vi "GetOneProperty.vi"() -> (0 "error out":errorcluster={"status"=TRUE, "code"=-375006, "source"="Unflatten From JSON in GetOneProperty.vi"}, 3 "setflag":string)   [LabVIEW 2019]
uses:
  <vilib>/httpClient/LabVIEWHTTPClient.lvlib
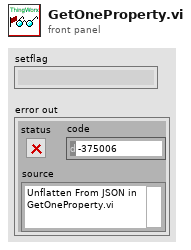
[diagram p1: front panel]
types:
  T1 = typedef "LabVIEWHTTPClient.lvlib/ClientHandle.ctl" = refnum<k1>
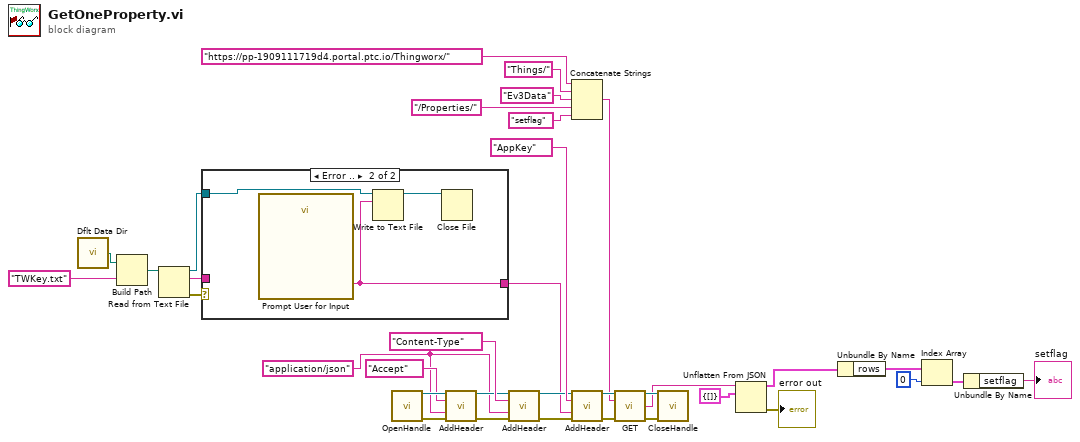
[diagram p0: block diagram]
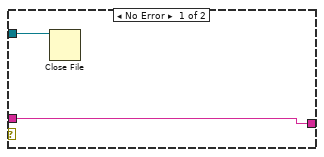
[diagram p2: hidden frame]
diagram:
  w14 = "application/json" ("value")
  n1 = call <vilib>:"Dflt Data Dir.vi"() -> ("App:Default Data Directory"=w7:path)
  n2 = Build Path(base path=w7, name or relative path="TWKey.txt") -> (appended path=w11:path)
  n3 = Read from Text File(file (use dialog)=w11) -> (refnum out=w8:refnum<file>, text=w10:string, error out=w12:errorcluster)  [unwired: 3 in, 1 out]
  n4 = case shown="Error .." w12 {
    tunnel: w8 -> [w36 w40]
    tunnel: [w37 w39] -> w9
    tunnel: w10 -> [w37 _]
    frame No Error {
      n5 = Close File(refnum=w36) -> ()  [unwired: 1 in, 2 out]
    }
    frame Error {
      n6 = call "Prompt User for Input"() -> ("key"=w39:string)  [unwired: 17 in, 2 out]
      n7 = Write to Text File(file (use dialog)=w40, text=w39) -> (refnum out=w38:refnum<file>)  [unwired: 2 in, 2 out]
      n8 = Close File(refnum=w38) -> ()  [unwired: 1 in, 2 out]
    }
  }
  n9 = call <vilib>:"OpenHandle.vi"() -> ("client handle out"=w34:T1, "error out"=w27:errorcluster)  [unwired: 14 in]
  n10 = call <vilib>:"AddHeader.vi"("client handle"=w34, "header"="Accept", "value"=w14, "error in (no error)"=w27) -> ("client handle out"=w30:T1, "error out"=w26:errorcluster)  [unwired: 10 in]
  n11 = call <vilib>:"AddHeader.vi"("client handle"=w30, "header"="Content-Type", "value"=w14, "error in (no error)"=w26) -> ("client handle out"=w29:T1, "error out"=w25:errorcluster)  [unwired: 10 in]
  n12 = Concatenate Strings("https://pp-1909111719d4.portal.ptc.io/Thingworx/" ("urlBase"), "Things/", "Ev3Data" ("Things"), "/Properties/", "setflag" ("service")) -> (w17:string)
  n13 = call <vilib>:"AddHeader.vi"("client handle"=w29, "header"="AppKey", "value"=w9, "error in (no error)"=w25) -> ("client handle out"=w28:T1, "error out"=w24:errorcluster)  [unwired: 10 in]
  n14 = call <vilib>:"GET.vi"("client handle"=w28, "url"=w17, "error in (no error)"=w24) -> ("client handle out"=w35:T1, "body"=w16:string, "error out"=w23:errorcluster)  [unwired: 9 in, 1 out]
  n15 = call <vilib>:"CloseHandle.vi"("client handle"=w35, "error in (no error)"=w23) -> ()  [unwired: 13 in, 1 out]
  n16 = Unflatten From JSON(JSON string=w16, type and defaults=cluster{"rows":cluster{"setflag":string}[]} {"rows"=[]}) -> (value=w6:cluster{"rows":cluster{"setflag":string}[]}, error out=→"error out":errorcluster)  [unwired: 5 in]
  n17 = Unbundle By Name(w6) -> ("rows"=w4:cluster{"setflag":string}[])
  n18 = Index Array(array=w4, index=0) -> (element=w2:cluster{"setflag":string})
  n19 = Unbundle By Name(w2) -> ("setflag"=→"setflag":string)
